vi "Log Data.vi"(8 "error in":errorcluster, 10 "Data":dbl[](array[numeric]), 11 "TDMS in":refnum<class "TDMS.lvclass">) -> (0 "error out":errorcluster, 3 "TDMS out":refnum<class "TDMS.lvclass">)   [LabVIEW 2019, in "ManejoArchivos.lvlib" / "TDMS.lvclass"]
uses:
  TDMS.lvclass
  C:/GitClones/PowerElectronics/28 Mayo Prueba Plantilla/Libraries/ManejoArchivos/Class Definitions/File/File.lvclass
  TDMS.lvclass/TDMS.ctl
  File/File.lvclass/File.ctl
  Read tdms file ref.vi
  File/Read Column Headers.vi
  File/Read Save Timestamp.vi
  Write tdms file ref.vi
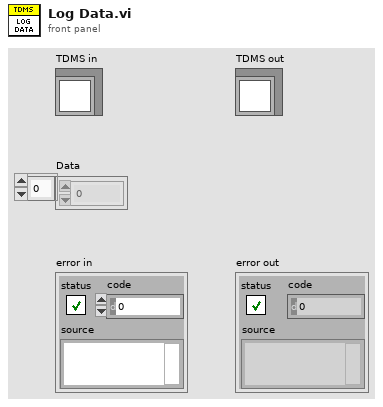
[diagram p1: front panel]
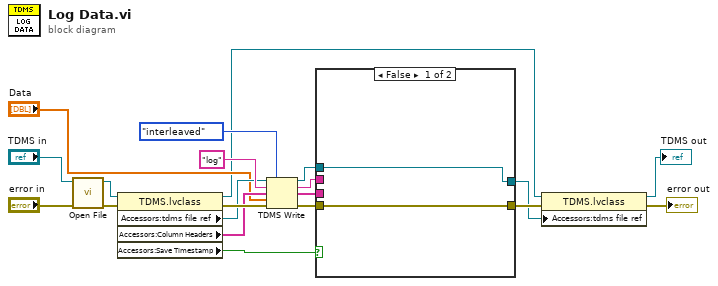
[diagram p0: block diagram]
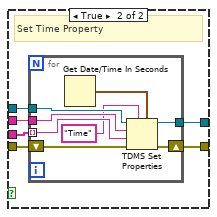
[diagram p2: hidden frame]
diagram:
  n1 = call-dynamic "Open File.vi"("error in"="error in", "TDMS in"="TDMS in") -> ("error out"=w7:errorcluster, "TDMS out"=w5:refnum<class "TDMS.lvclass">)  [unwired: 8 in]
  n2 = property class="TDMS.lvclass"(reference=w5, error in=w7) -> (reference out=w3:refnum<class "TDMS.lvclass">, error out=w18:errorcluster, "Accessors:tdms file ref"=w11:refnum<k34>, "Accessors:Column Headers"=w10:string[], "Accessors:Save Timestamp"=w8:bool)
  n3 = TDMS Write(0:w11, 1:enum16{"decimated", "interleaved"}."interleaved" ("data layout (0:decimated)"), 5:"log" ("group name in (Untitled)"), 7:w10, 9:"Data", 11:w18) -> (4:w14:refnum<k34>, 6:w13:string, 8:w12:string[], 15:w19:errorcluster)
  n4 = case shown="False" w8 {
    tunnel: w14 -> [w21 w26]
    tunnel: w19 -> [w22 w28]
    tunnel: [w22 w27] -> w17
    tunnel: w13 -> [_ w25]
    tunnel: w12 -> [_ w24]
    tunnel: [w21 w23] -> w1
    frame False {
    }
    frame True {
      # "Set Time Property"
      n5 = for {
        tunnel: w25 -> [w32]
        shift-right: [w35] -> w27
        shift-left: w28 -> [w36]
        tunnel: w24 -> [w31] mode=indexing
        tunnel: w26 -> [w34]
        tunnel: [w33] -> w23
        n6 = Get Date/Time In Seconds() -> (seconds since 1Jan1904=w29:timestamp)
        n7 = TDMS Set Properties(5:w29, 7:"Time", 8:w36, 9:w31, 10:w32, 11:w34) -> (0:w35:errorcluster, 3:w33:refnum<k34>)  [unwired: 2 out]
      }
    }
  }
  n8 = property class="TDMS.lvclass"(reference=w3, error in=w17, "Accessors:tdms file ref"=w1) -> (reference out=→"TDMS out":refnum<class "TDMS.lvclass">, error out=→"error out":errorcluster)
